vi "Area of Triangle.vi"(1 "Side C (cm)":dbl, 2 "Side B (cm)":dbl, 3 "Side A (cm)":dbl) -> (0 "Area of Triangle (cm^2)":dbl)   [LabVIEW 2013]
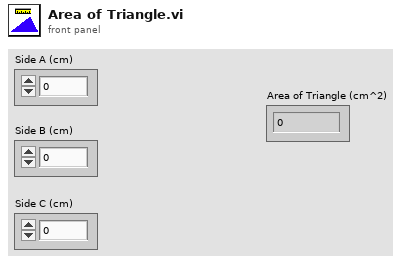
[diagram p1: front panel]
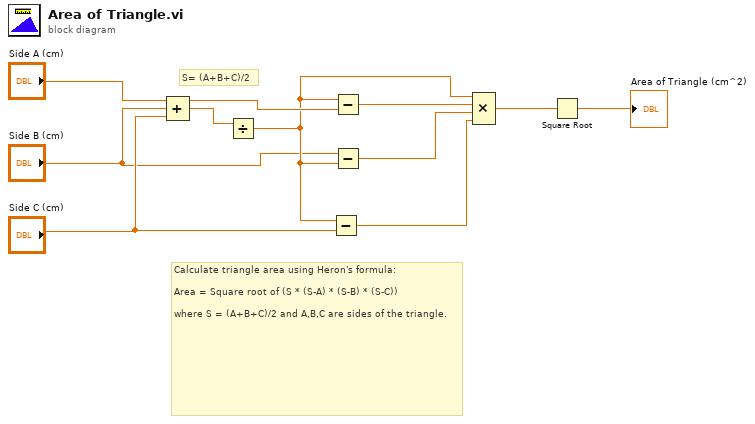
[diagram p0: block diagram]
diagram:
  # "S= (A+B+C)/2"
  # "Calculate triangle area using Heron's formula:\n\nArea = Square root of (S * (S-A) * (S-B) * (S-C))\n\nwhere S = (A+B+C)/2 and A,B,C are sides of the triangle."
  n1 = Compound Arithmetic op=ADD("Side A (cm)", "Side B (cm)", "Side C (cm)") -> (w3:dbl)
  n2 = Divide(x=w3) -> (x/y=w2:dbl)  [unwired: 1 in]
  n3 = Subtract(x=w2, y="Side C (cm)") -> (x-y=w6:dbl)
  n4 = Subtract(x=w2, y="Side A (cm)") -> (x-y=w8:dbl)
  n5 = Subtract(x="Side B (cm)", y=w2) -> (x-y=w7:dbl)
  n6 = Compound Arithmetic op=MULTIPLY(w2, w8, w7, w6) -> (w5:dbl)
  n7 = Square Root(x=w5) -> (sqrt(x)=→"Area of Triangle (cm^2)":dbl)
